vi "Test 2.vi"() -> ()   [LabVIEW 2016, in "Drona Path obtn.lvlib"]
doc: "This Test is used to check for drona path if the control is present inside a subpanel"
uses:
  Drona Path obtn.lvlib
  Typedefs/Test LV2 Enum.ctl
panel:
  out "Drona Path":string
  out "error out":errorcluster
  in  "error in (no error)":errorcluster
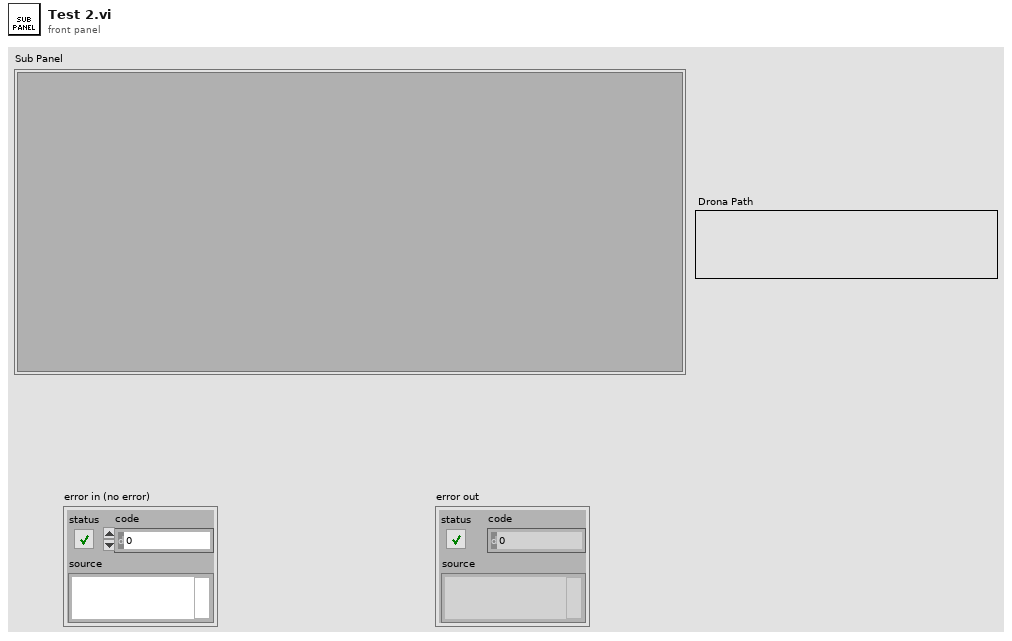
[diagram p1: front panel]
types:
  T1 = typedef "Drona Path obtn.lvlib/Test LV2 Enum.ctl" = enum16{"Initialize", "Write", "Read"}
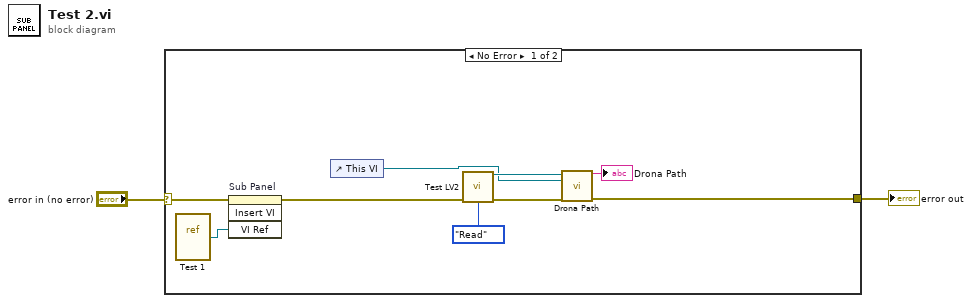
[diagram p0: block diagram]
diagram:
  n1 = case shown="No Error" "error in (no error)" {
    selector: "error in (no error)" -> [w9 w12]
    tunnel: [w10 w12] -> w1
    frame No Error {
      n2 = vi-ref "Test 1.vi"() -> (w4:refnum<vi>)
      n3 = invoke on="Sub Panel" class="SubPnl" method="Insert VI"(error in=w9, "VI Ref"=w4) -> (error out=w8:errorcluster)  [unwired: 2 in, 3 out]
      n4 = control-ref of="This VI"() -> (w3:refnum<vi>)
      n5 = call "Test LV2.vi"("error in (no error)"=w8, "Operation"=Test_LV2_Enum."Read") -> ("Ref Out"=w6:refnum<vi>, "error out"=w11:errorcluster)  [unwired: 12 in]
      n6 = call "Drona Path.vi"("Control reference"=w6, "Active VI reference"=w3, "error in (no error)"=w11) -> ("Drona Path"=→"Drona Path":string, "error out"=w10:errorcluster)  [unwired: 11 in]
    }
    frame Error {
    }
  }
  "error out" <- w1
